vi "WS1050 VSA_Delta C Calculation.vi"(8 "error in (no error)":errorcluster, 10 "CAP_T":string[](array[string]), 11 "CAP_T0":string[](array[string])) -> (0 "error out":errorcluster, 2 "Delta C(pF)":dbl[](array[numeric]), 3 "Delta C(pF)":string[](array[string]))   [LabVIEW 2012]
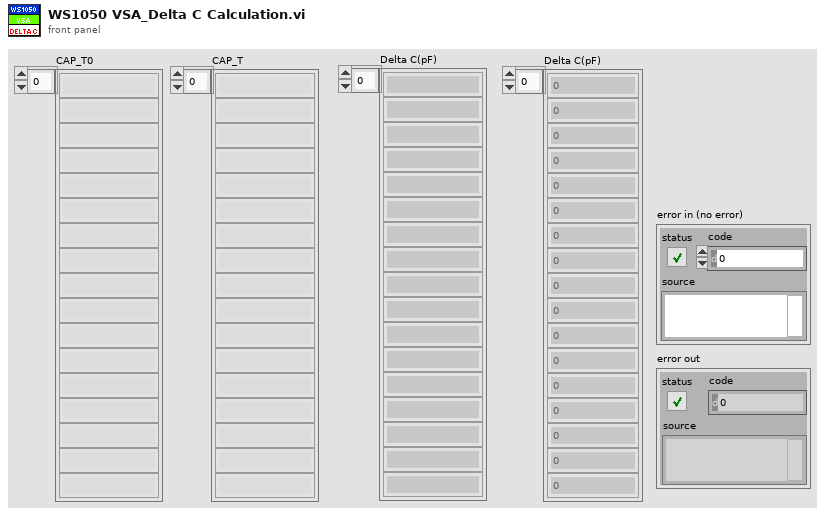
[diagram p1: front panel]
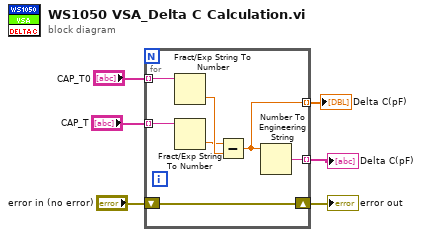
[diagram p0: block diagram]
diagram:
  n1 = for {
    tunnel: "CAP_T0" -> [w8] mode=indexing
    tunnel: "CAP_T" -> [w7] mode=indexing
    tunnel: [w10] -> w4 mode=indexing
    tunnel: [w9] -> w1 mode=indexing
    shift-right: [w13] -> w5
    shift-left: "error in (no error)" -> [w13]
    n2 = Fract/Exp String To Number(string=w8) -> (number=w12:dbl)  [unwired: 3 in, 1 out]
    n3 = Fract/Exp String To Number(string=w7) -> (number=w11:dbl)  [unwired: 3 in, 1 out]
    n4 = Subtract(x=w11, y=w12) -> (x-y=w9:dbl)
    n5 = Number To Engineering String(4:w9) -> (0:w10:string)  [unwired: 3 in]
  }
  "error out" <- w5
  "Delta C(pF)" <- w4
  "Delta C(pF)" <- w1
